vi "_save_csv_InPhaseStep_only.vi"(7 "delimiter (\\t)":string="SingleCh_", 11 "dataInput":string[][](array[string])) -> (3 "FileName":string)   [LabVIEW 2023]
uses:
  <vilib>/Utility/file.llb/Write Delimited Spreadsheet (string).vi
panel:
  out "appended path":path
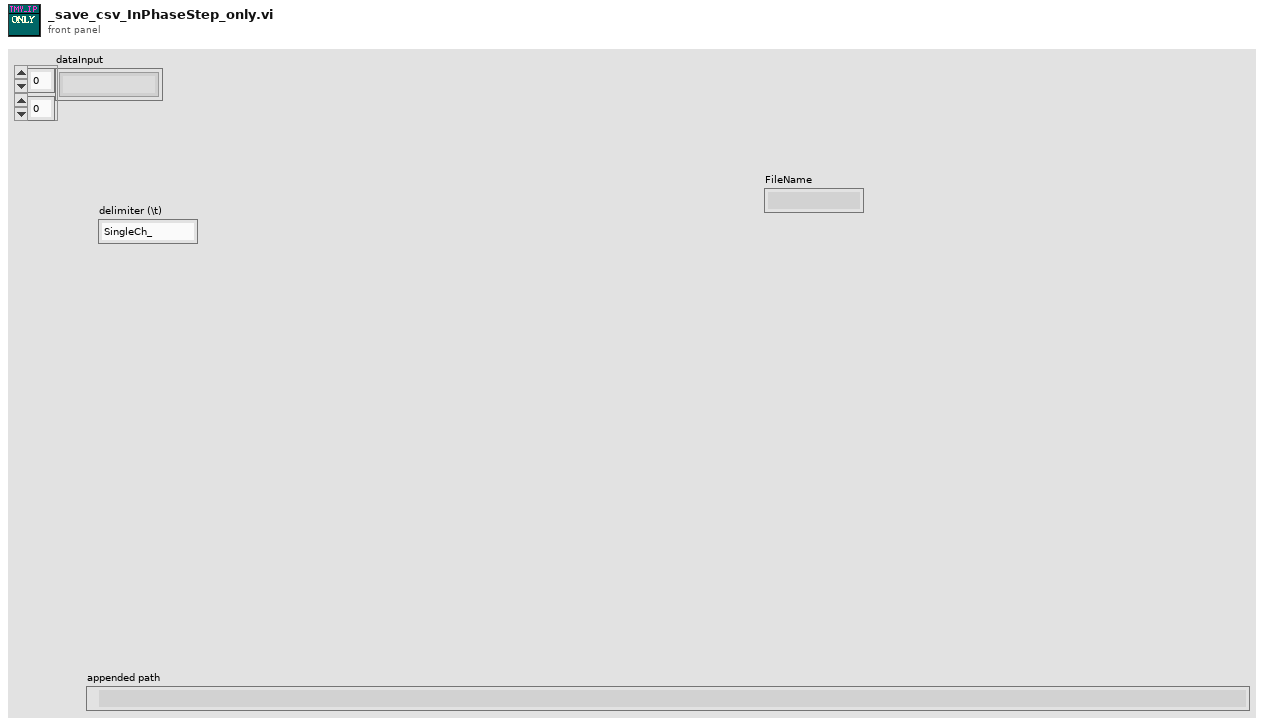
[diagram p1: front panel]
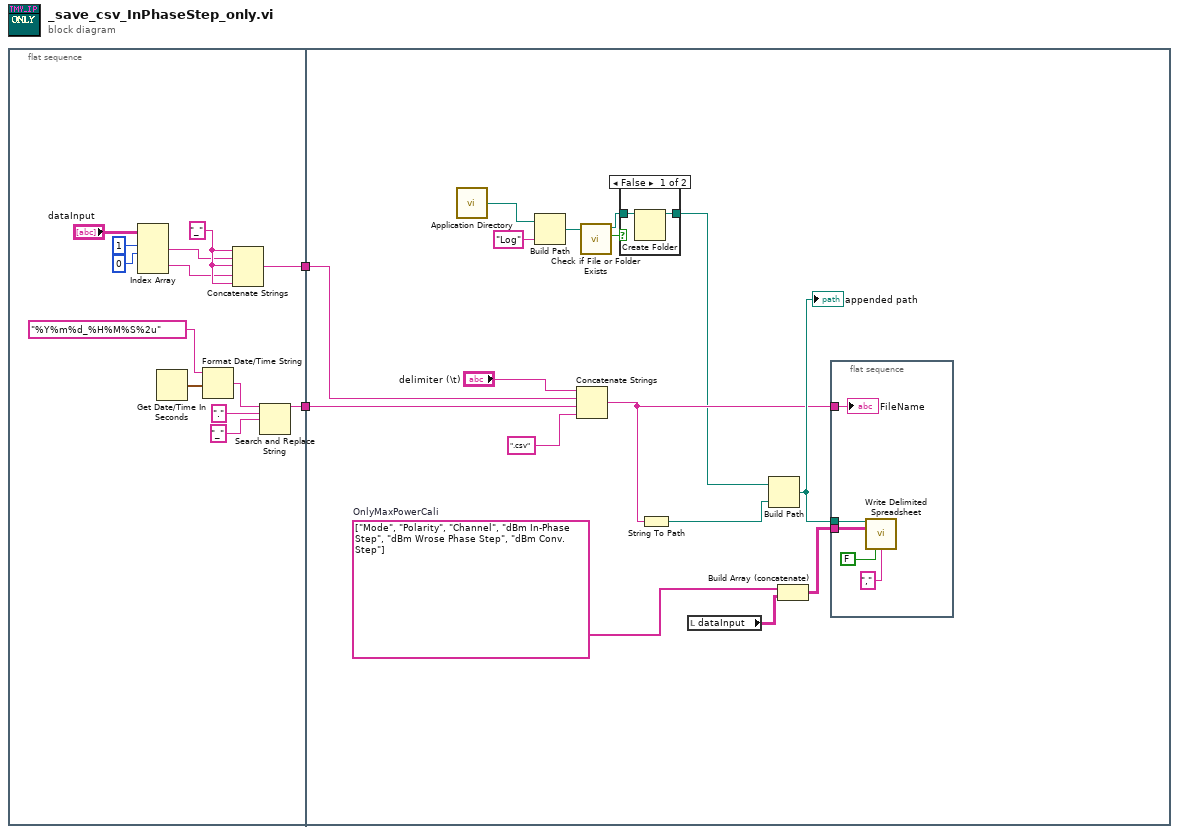
[diagram p0: block diagram]
diagram:
  n1 = flat-sequence {
    tunnel: [w10] -> w2
    tunnel: [w3] -> w1
    tunnel: w2 -> [w23]
    tunnel: w1 -> [w21]
    frame #0 {
      w6 = "_"
      n2 = Index Array(array="dataInput", index (row) #1=1 ("index (row)"), index (col) #1=0 ("disabled index (col)")) -> (element #1=w5:string, element #2=w4:string)  [unwired: 2 in]
      n3 = Get Date/Time In Seconds() -> (seconds since 1Jan1904=w15:timestamp)
      n4 = Format Date/Time String(time format string (%c)="%Y%m%d_%H%M%S%2u", seconds (now)=w15) -> (date/time string=w13:string)  [unwired: 1 in]
      n5 = Concatenate Strings(w6, w5, w6, w4, w6) -> (w3:string)
      n6 = Search and Replace String(input string=w13, search string=".", replace string="_") -> (result string=w10:string)  [unwired: 5 in, 3 out]
    }
    frame #1 {
      w27 = string[] ["Mode", "Polarity", "Channel", "dBm In-Phase Step", "dBm Wrose Phase Step", "dBm Conv. Step"]  # OnlyMaxPowerCali
      n7 = call <vilib>:"Application Directory.vi"() -> ("Application Directory"=w25:path)
      n8 = Build Path(base path=w25, name or relative path="Log") -> (appended path=w17:path)
      n9 = Concatenate Strings("delimiter (\\t)", w21, w23, ".csv" ("delimiter (\\t)")) -> (w28:string)
      n10 = call <vilib>:"Check if File or Folder Exists.vi"("path"=w17) -> ("file or folder exists?"=w19:bool, "dup path"=w18:path)  [unwired: 8 in, 1 out]
      n11 = case shown="False" w19 {
        tunnel: w18 -> [w33 w34]
        tunnel: [w32 w34] -> w16
        frame False {
          n12 = Create Folder(path (use dialog)=w33) -> (created path=w32:path)  [unwired: 2 in, 2 out]
        }
        frame True {
        }
      }
      n13 = String To Path(string=w28) -> (path=w30:path)
      n14 = local read "dataInput"() -> (w20:string[][])
      n15 = Build Path(base path=w16, name or relative path=w30) -> (appended path=w29:path)
      "appended path" <- w29
      n16 = Build Array (concatenate)(w27, w20) -> (w26:string[][])
      n17 = flat-sequence {
        tunnel: w29 -> [w38]
        tunnel: w28 -> [w36]
        tunnel: w26 -> [w35]
        frame #0 {
          n18 = call-poly <vilib>:"Write Delimited Spreadsheet.vi"("file path (dialog if empty)"=w38, "2D data"=w35, "transpose? (no:F)"=FALSE, "delimiter (\\t)"="," ("delimiter (\\t)")) -> ()  [unwired: 10 in, 2 out]
          "FileName" <- w36
        }
      }
    }
  }
